vi "Synchio.PushPull.vi"(8 "error in (no error)":errorcluster, 10 "IO Info":T1={"AI task"=["", ""], "sampling info"={"Fs"=1000.0, "#s"=1000.0}, "AO Array"=[], "AO Task"=[], "Reset"=FALSE} {"sampling info"."Fs" format="%.2p"}, 11 "SynchIO in":refnum<class "SynchIO.lvclass">) -> (0 "error out":errorcluster, 2 "Input Signals":waveform(dbl)[](array[waveform]), 3 "SynchIO out":refnum<class "SynchIO.lvclass">)   [LabVIEW 2016, in "SynchIO.lvclass"]
uses:
  SynchIO.lvclass
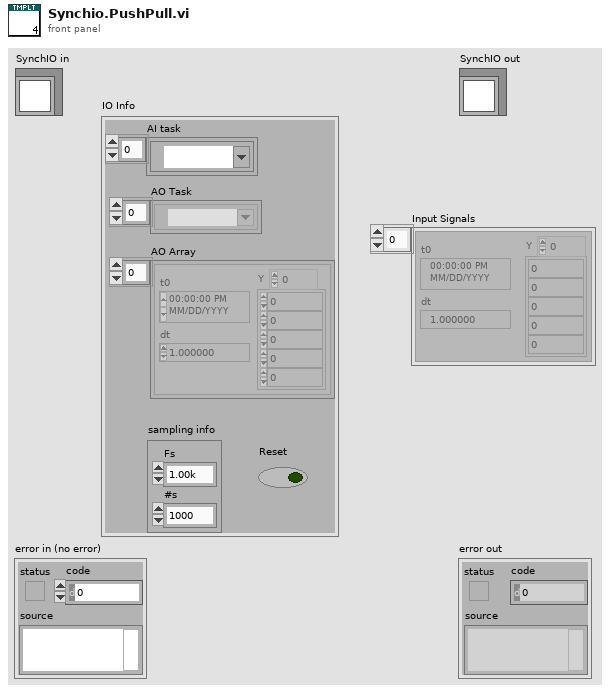
[diagram p1: front panel]
types:
  T1 = cluster{"AI task":refnum<k21>[], "sampling info":cluster{"Fs":dbl, "#s":dbl}, "AO Array":waveform(dbl)[], "AO Task":refnum<k21>[], "Reset":bool}
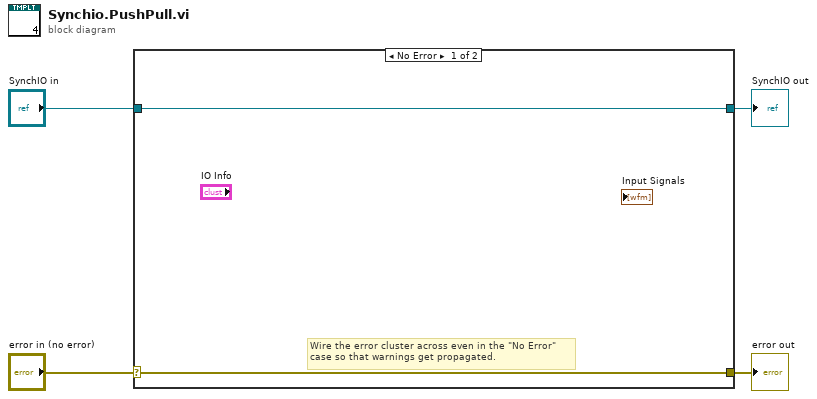
[diagram p0: block diagram]
diagram:
  n1 = case shown="No Error" "error in (no error)" {
    selector: "error in (no error)" -> [w5 w8]
    tunnel: [w5 w8] -> w3
    tunnel: [w6 w7] -> w1
    tunnel: "SynchIO in" -> [w6 w7]
    frame No Error {
      # "Wire the error cluster across even in the \"No Error\"\ncase so that warnings get propagated."
    }
    frame Error {
    }
  }
  "error out" <- w3
  "SynchIO out" <- w1
